vi "Execute.vi"(8 "error in":errorcluster, 11 "Plugin_Controller in":refnum<class "Plugin_Controller.lvclass">) -> (0 "error out":errorcluster, 3 "Plugin_Controller out":refnum<class "Plugin_Controller.lvclass">)   [LabVIEW 2020, in "Plugin.lvlib" / "Plugin_Controller.lvclass"]
doc: "Executes the output channel configuration and reads the measurement data from input channels."
uses:
  Plugin_Controller.lvclass
  Plugin_Controller.lvclass/Plugin_Controller.ctl
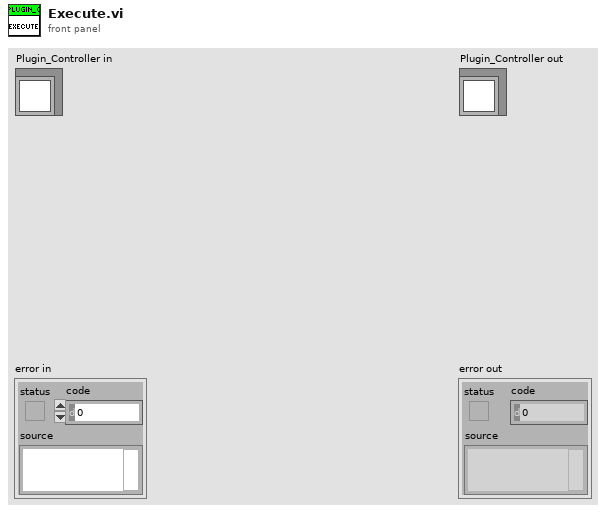
[diagram p1: front panel]
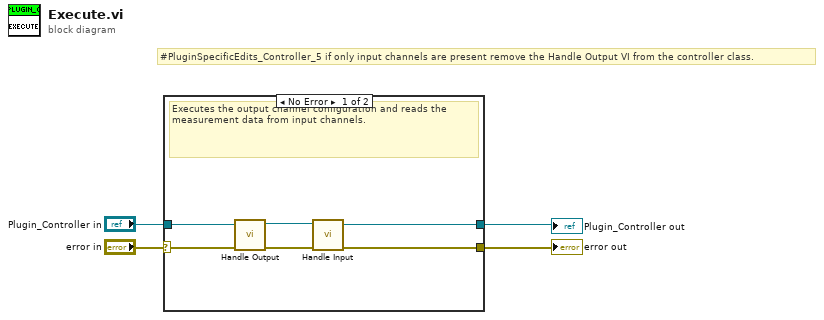
[diagram p0: block diagram]
diagram:
  # "#PluginSpecificEdits_Controller_5 if only input channels are present remove the Handle Output VI from the controller class."
  n1 = case shown="No Error" "error in" {
    selector: "error in" -> [w6 w12]
    tunnel: [w5 w12] -> w3
    tunnel: [w8 w11] -> w1
    tunnel: "Plugin_Controller in" -> [w9 w11]
    frame No Error {
      # "Executes the output channel configuration and reads the measurement data from input channels."
      n2 = call "Handle Output.vi"("error in"=w6, "Plugin_Controller in"=w9) -> ("error out"=w7:errorcluster, "Plugin_Controller out"=w10:refnum<class "Plugin_Controller.lvclass">)  [unwired: 8 in]
      n3 = call "Handle Input.vi"("error in (no error)"=w7, "Plugin_Controller in"=w10) -> ("error out"=w5:errorcluster, "Plugin_Controller out"=w8:refnum<class "Plugin_Controller.lvclass">)  [unwired: 8 in]
    }
    frame Error {
    }
  }
  "error out" <- w3
  "Plugin_Controller out" <- w1
